vi "Drive Controller.vi"(8 "error in":errorcluster) -> ()   [LabVIEW 2018]
doc: "This VI executes continuously carrying out the current operation and responding to updates or new operation requests. It will often contain the timing or control code that is difficult to place directly in TeleOp. This VI generally opens all sensors and motors and isolates the rest of the robot code from knowing implementation details of how the operations are carried out."
uses:
  <vilib>/Rock Robotics/WPI/Framework/Completion Status.ctl
  Drive Setpoints.ctl
  Drive Operations.ctl
  <vilib>/Rock Robotics/SystemInterfaces/DIO/FPGA_DIOPWMChannel.ctl
  <vilib>/Rock Robotics/WPI/DriverStation/WPI_DriverStationRobotMode2.ctl
  <vilib>/Rock Robotics/WPI/RobotDrive/WPI_RobotDriveOpen4MotorWithJaguar.vi
  Framework/Robot Global Data.vi
  <vilib>/Rock Robotics/WPI/ThirdParty/Sensors/navX/_Processing Loop/FRIC_navX_Internal_SPI_ProcessingLoop.vi
panel:
  in  "Reset Gyro":bool
  in  "navX  start":dbl
  in  "Angle":dbl
  in  "Interactive Values":T1
  in  "Buttons":cluster{"Execute Cmd":bool, "Abort Cmd":bool}
  out "Command Timing":cluster{"Start Time (ms)":u32, "Iterations":i32}
  out "Status":T3
  out "Setpoints":T4(graph)
  out "Current\nCmd":string
  # "Tip: The graph shows the motor setpoints. It may also be helpful to observe inputs and sensor values.\nYou may also want to display tuning or debugging controls."
  # "Interactive Command: You may fill in the settings for a command\nand schedule it with the Execute button. You can observe and abort\nany command while fine tuning the code for the controller."
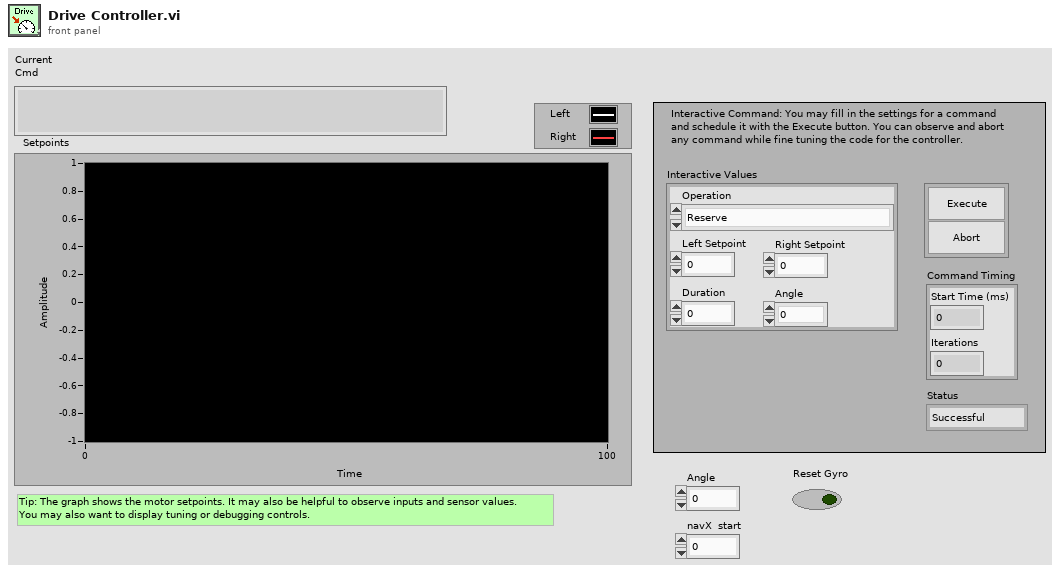
[diagram p1: front panel]
types:
  T1 = typedef "Drive Setpoints.ctl" = cluster{"Operation":T2, "Left Setpoint":dbl, "Right Setpoint":dbl, "Duration":dbl, "Angle":dbl}
  T2 = typedef "Drive Operations.ctl" = enum16{"Reserve", "Read Current", "Immediate", "Drive for Time", "Drive for Distance", "Turn to Angle"}
  T3 = typedef "Completion Status.ctl" = enum16{"Successful", "Aborted", "Incomplete"}
  T4 = cluster{"Left Setpoint":dbl, "Right Setpoint":dbl}
  T5 = typedef "FPGA_DIOPWMChannel.ctl" = enum8{"PWM 0", "PWM 1", "PWM 2", "PWM 3", "PWM 4", "PWM 5", "PWM 6", "PWM 7", "PWM 8", "PWM 9", "PWM MXP 0", "PWM MXP 1", "PWM MXP 2", "PWM MXP 3", "PWM MXP 4", "PWM MXP 5", "PWM MXP 6", "PWM MXP 7", "PWM MXP 8", "PWM MXP 9", "Invalid"}
  T6 = typedef "WPI_RobotDriveDevRef.ctl" = cluster{"DevStatus":errorcluster, "Motors[]":T7[], "Square Inputs":bool, "Max Output":dbl}
  T7 = typedef "WPI_MotorControlDeviceRef.ctl" = cluster{"DeviceStatus":errorcluster, "Type":T8, "PWM":cluster{"PWM Channel":T5, "DeadBand":T9}, "CAN":cluster{"Device Number":u8, "SetOutput VI Ref":variant, "GetOutput VI Ref":variant, "Enable VI Ref":variant, "Disable VI Ref":variant, "Data":variant}, "Invert":bool, "DIO PWM":cluster{"PWM \"Enable\" Channel":T5, "DIOChannel":T10, "PWM Rate":dbl}}
  T8 = typedef "WPI_MotorControlType.ctl" = enum16{"PWM", "CAN", "DIO PWM"}
  T9 = typedef "WPI_PWMDeadband.ctl" = cluster{"Name":string, "maxPositivePwm":i32, "minPositivePwm":i32, "centerPwm":i32, "maxNegativePwm":i32, "minNegativePwm":i32, "angularRange":u16}
  T10 = typedef "FPGA_DIOChannel.ctl" = enum8{"DIO 0", "DIO 1", "DIO 2", "DIO 3", "DIO 4", "DIO 5", "DIO 6", "DIO 7", "DIO 8", "DIO 9", "DIO MXP 0", "DIO MXP 1", "DIO MXP 2", "DIO MXP 3", "DIO MXP 4", "DIO MXP 5", "DIO MXP 6", "DIO MXP 7", "DIO MXP 8", "DIO MXP 9", "DIO MXP 10", "DIO MXP 11", "DIO MXP 12", "DIO MXP 13", "DIO MXP 14", "DIO MXP 15", "SPI Port CS1", "SPI Port CS2", "SPI Port CS3", "SPI Port MISO", "SPI Port MOSI", "Invalid"}
  T11 = typedef "Command Status Info.ctl" = cluster{"Name":string, "Status":T3, "notifier out":T12}
  T12 = typedef "Completion Notifier.ctl" = refnum<notifier>
  T13 = cluster{"SubSystem Data":T1, cluster{"Start Time (ms)":u32, "Iterations":i32}, cluster{"Command Info":T11, "Description":string, "Default Command":T1, "queue out":refnum<queue>, "Subsystem Name":string}}
  T14 = typedef "WPI_DriverStationRobotMode2.ctl" = enum16{"Autonomous Disabled", "Autonomous Enabled", "Teleop Disabled", "Teleop Enabled", "Disconnected", "Finish", "Test Disabled", "Test Enabled", "Emergency Stopped"}
  T15 = cluster{"Yaw":dbl, "Roll":dbl, "Pitch":dbl, "Heading":dbl, "Fused Heading":dbl}
  T16 = cluster{"SubSystem Data":T1, cluster{"Start Time (ms)":u32, "Iterations":i32}, "Default Command Arguments":cluster{"Command Info":T11, "Description":string, "Default Command":T1, "queue out":refnum<queue>, "Subsystem Name":string}}
  T17 = cluster{"Don't move motors while reserved":dbl, "Don't move motors while reserved":dbl}
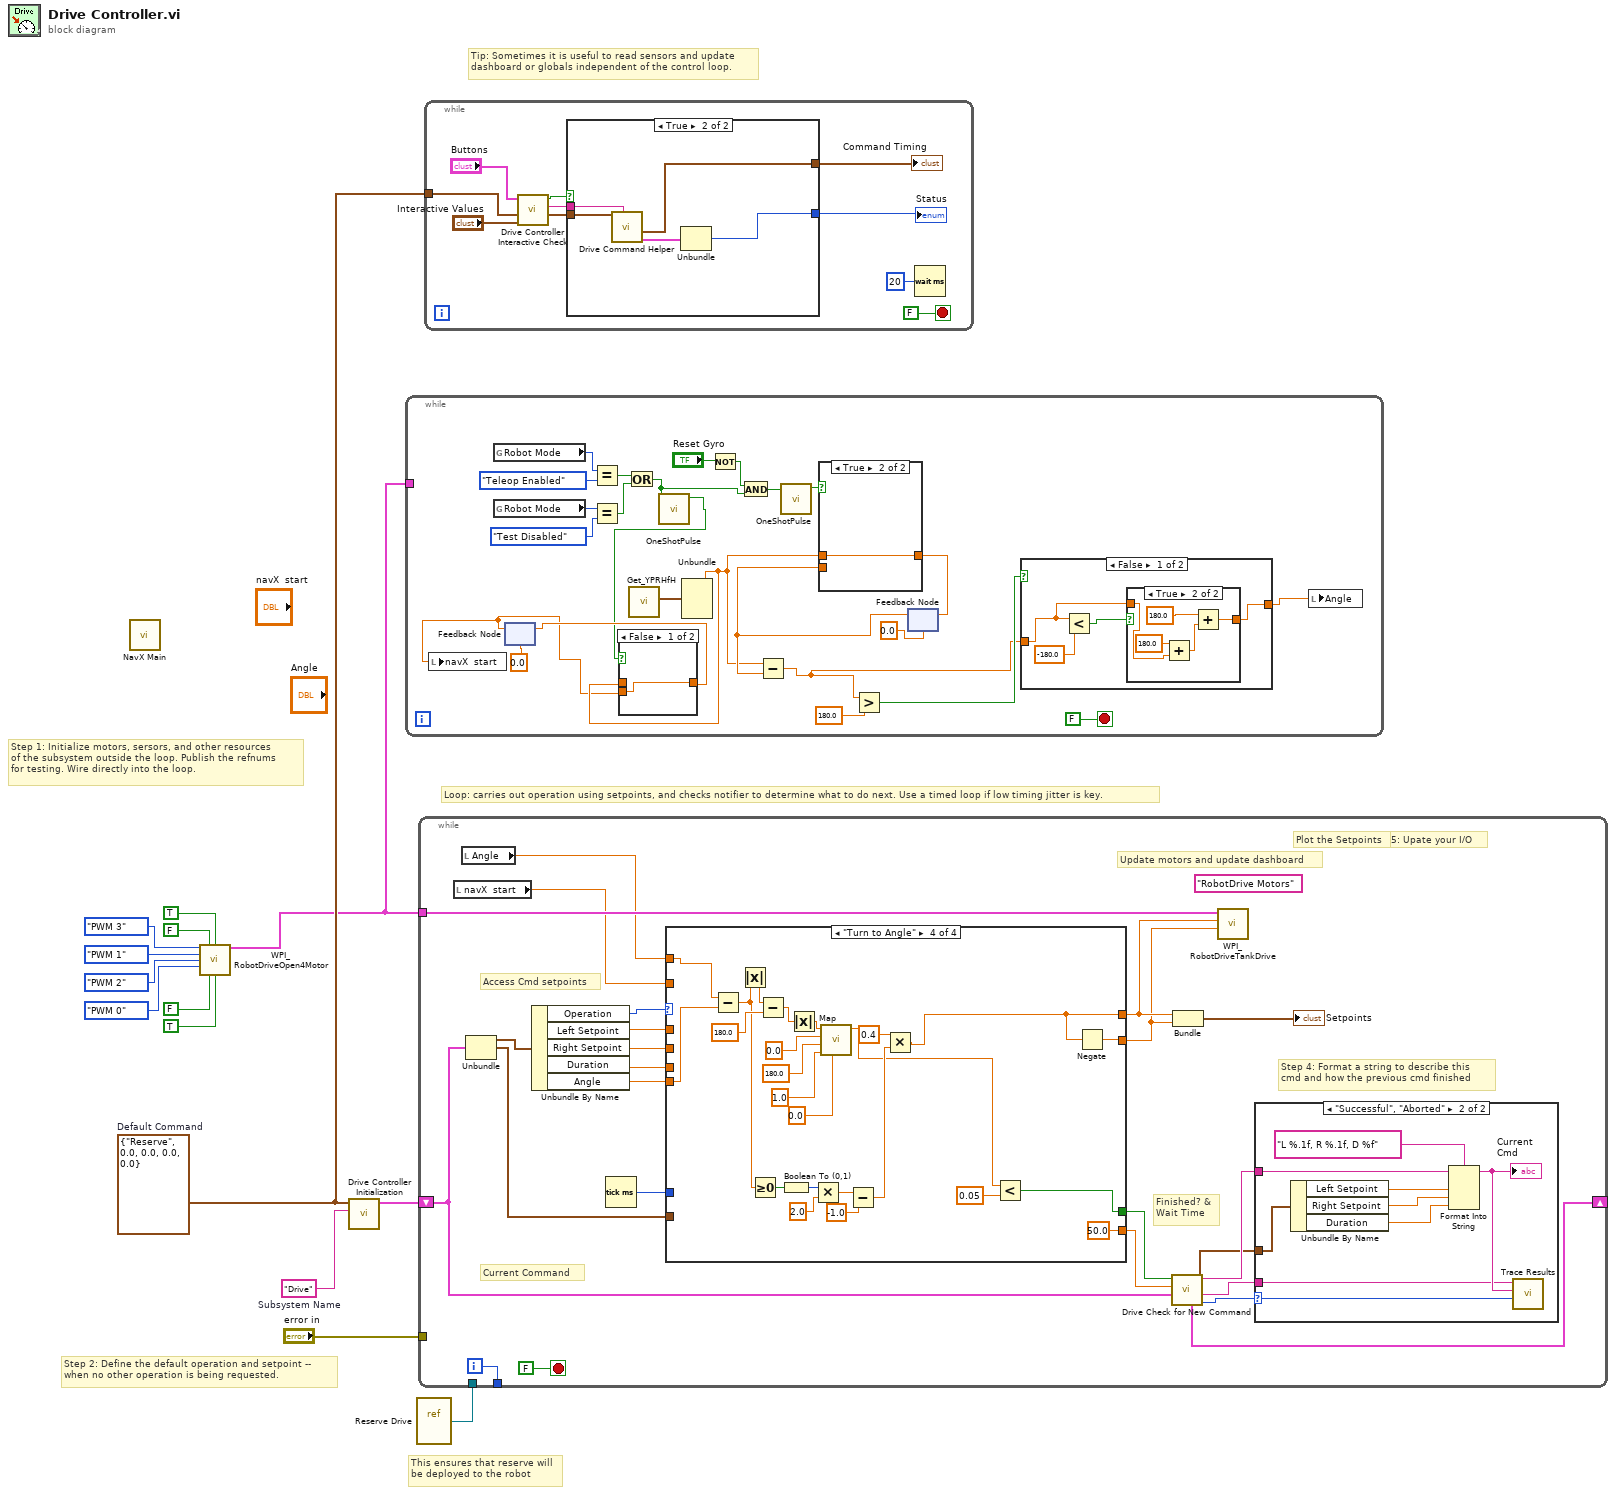
[diagram p0: block diagram]
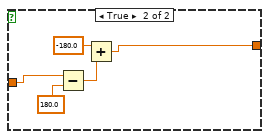
[diagram p3: hidden frame]
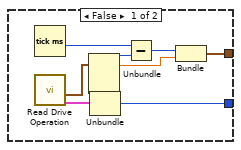
[diagram p6: hidden frame]
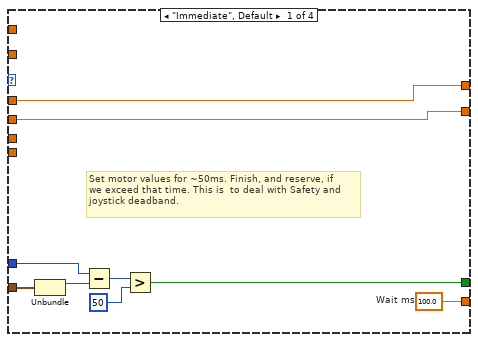
[diagram p8: hidden frame]
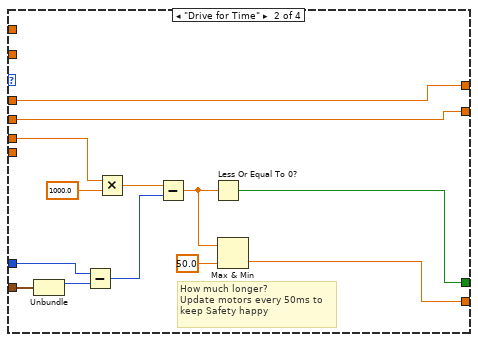
[diagram p9: hidden frame]
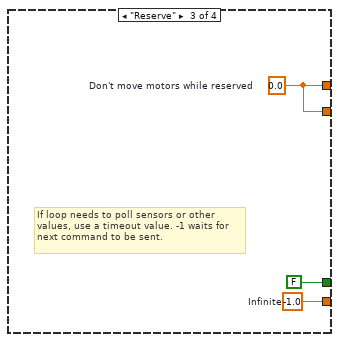
[diagram p10: hidden frame]
diagram:
  w10 = T1 {"Operation"=enum."Reserve", "Left Setpoint"=0.0, "Right Setpoint"=0.0, "Duration"=0.0, "Angle"=0.0}  # Default Command
  w14 = "Drive"  # Subsystem Name
  # "This ensures that reserve will\nbe deployed to the robot"
  # "Tip: Sometimes it is useful to read sensors and update\ndashboard or globals independent of the control loop."
  # "Step 2: Define the default operation and setpoint --\nwhen no other operation is being requested."
  # "Step 1: Initialize motors, sersors, and other resources\nof the subsystem outside the loop. Publish the refnums\nfor testing. Wire directly into the loop."
  # "Loop: carries out operation using setpoints, and checks notifier to determine what to do next. Use a timed loop if low timing jitter is key."
  n1 = call-poly <vilib>:"NavX Main.vi"() -> ()  [unwired: 12 in]
  n2 = call-poly <vilib>:"WPI_RobotDriveOpen4Motor.vi"("Rear Left Motor"=FPGA_DIOPWMChannel."PWM 3", "Rear Left Motor Inverted"=FALSE, "Rear Right Motor Inverted"=TRUE, "Rear Right Motor"=FPGA_DIOPWMChannel."PWM 1", "Front Left Motor"=FPGA_DIOPWMChannel."PWM 2", "Front Right Motor"=FPGA_DIOPWMChannel."PWM 0", "Front Left Motor Inverted"=FALSE, "Front Right Motor Inverted"=TRUE) -> ("RobotDriveDevRef"=w1:T6)  [unwired: 6 in, 1 out]
  n3 = call "Drive Controller Initialization.vi"("Subsystem Name"=w14, "Default Command"=w10) -> ("Current Command"=w12:T13)  [unwired: 9 in]
  n4 = while {
    tunnel: w1 -> [_]
    stop <- FALSE stop-if-true
    n5 = global read "Robot Global Data.vi" "Robot Mode"() -> (w35:T14)
    n6 = global read "Robot Global Data.vi" "Robot Mode"() -> (w37:T14)
    n7 = feedback #1(0.0) -> (w25:dbl)
    n8 = local write "navX  start"(w25) -> ()
    n9 = Equal?(x=w35, y=WPI_DriverStationRobotMode2."Teleop Enabled") -> (x = y?=w33:bool)
    n10 = Equal?(x=w37, y=WPI_DriverStationRobotMode2."Test Disabled") -> (x = y?=w32:bool)
    n11 = Or(x=w33, y=w32) -> (x .or. y?=w19:bool)
    n12 = call <vilib>:"Get_YPRHfH.vi"() -> ("YRPHfH"=w38:T15)  [unwired: 11 in]
    n13 = call "OneShotPulse.vi"("Input"=w19) -> ("Output"=w24:bool)  [unwired: 10 in]
    n14 = Unbundle(w38) -> ("Yaw"=w27:dbl)  [unwired: 4 out]
    n15 = case shown="False" w24 {
      tunnel: w27 -> [_ w56]
      tunnel: [w55 w56] -> w26
      tunnel: w25 -> [w55 _]
      frame False {
      }
      frame True {
      }
    }
    n16 = feedback-in #1(w26) -> ()
    n17 = Not(x="Reset Gyro") -> (.not. x?=w20:bool)
    n18 = And(x=w20, y=w19) -> (x .and. y?=w22:bool)
    n19 = call "OneShotPulse.vi"("Input"=w22) -> ("Output"=w23:bool)  [unwired: 10 in]
    n20 = feedback #2(0.0 ("Yaw")) -> (w29:dbl)
    n21 = Subtract(x=w27, y=w29) -> (x-y=w15:dbl)
    n22 = case shown="True" w23 {
      tunnel: w27 -> [_ w58]
      tunnel: [w57 w58] -> w31
      tunnel: w29 -> [w57 _]
      frame False {
      }
      frame True {
      }
    }
    n23 = Greater?(x=w15, y=180.0) -> (0:w17:bool)
    n24 = feedback-in #2(w31) -> ()
    n25 = case shown="False" w17 {
      tunnel: [w40 w52] -> w16
      tunnel: w15 -> [w41 w50]
      frame False {
        n26 = Less?(x=w41, y=-180.0) -> (x < y?=w42:bool)
        n27 = case shown="True" w42 {
          tunnel: w41 -> [w44 w47]
          tunnel: [w44 w45] -> w40
          frame False {
          }
          frame True {
            n28 = Add(x=180.0, y=w47) -> (x+y=w46:dbl)
            n29 = Add(x=180.0, y=w46) -> (x+y=w45:dbl)
          }
        }
      }
      frame True {
        n30 = Subtract(x=w50, y=180.0) -> (x-y=w53:dbl)
        n31 = Add(x=-180.0, y=w53) -> (x+y=w52:dbl)
      }
    }
    n32 = local write "Angle"(w16) -> ()
  }
  n33 = vi-ref "Reserve Drive.vi"() -> (w11:refnum<vi>)
  n34 = while {
    shift-right: [w69] -> _
    shift-left: w12 -> [w62]
    tunnel: [w81] -> _
    tunnel: w1 -> [w77]
    tunnel: "error in" -> [_]
    tunnel: w11 -> [_]
    i -> [w81]
    stop <- FALSE stop-if-true
    (unwired) "RobotDrive Motors" ("Name")
    # "Step 5: Upate your I/O"
    # "Step 4: Format a string to describe this\ncmd and how the previous cmd finished"
    # "Current Command"
    # "Update motors and update dashboard"
    # "Plot the Setpoints"
    # "Access Cmd setpoints"
    # "Finished? &\nWait Time"
    n35 = local read "navX  start"() -> (w59:dbl)
    n36 = local read "Angle"() -> (w60:dbl)
    n37 = Unbundle(w62) -> ("SubSystem Data"=w76:T1, w63:cluster{"Start Time (ms)":u32, "Iterations":i32})  [unwired: 1 out]
    n38 = Unbundle By Name(w76) -> ("Operation"=w75:T2, "Left Setpoint"=w74:dbl, "Right Setpoint"=w73:dbl, "Duration"=w72:dbl, "Angle"=w61:dbl)
    n39 = Tick Count (ms)() -> (millisecond timer value=w71:u32)
    n40 = case shown="\"Turn to Angle\"" w75 {
      tunnel: [w100 w101 w116 50.0 ("Infinite")] -> w68
      tunnel: [w93 w108 FALSE ("ignore previous (F)") w138] -> w67
      tunnel: w63 -> [w92 w110 _ _]
      tunnel: [w99 w107 w114 w136] -> w79
      tunnel: [w98 w106 w114 w137] -> w78
      tunnel: w74 -> [w99 w107 _ _]
      tunnel: w73 -> [w98 w106 _ _]
      tunnel: w72 -> [_ w105 _ _]
      tunnel: w71 -> [w94 w104 _ _]
      tunnel: w60 -> [_ _ _ w118]
      tunnel: w61 -> [_ _ _ w135]
      tunnel: w59 -> [_ _ _ _]
      frame "Immediate", Default {
        w100 = 100.0  # Wait ms
        # "Set motor values for ~50ms. Finish, and reserve, if\nwe exceed that time. This is  to deal with Safety and\njoystick deadband."
        n41 = Unbundle(w92) -> ("Start Time (ms)"=w95:u32)  [unwired: 1 out]
        n42 = Subtract(x=w94, y=w95) -> (x-y=w96:u32)
        n43 = Greater?(x=w96, y=u8 50 ("Left Motor")) -> (0:w93:bool)
      }
      frame "Drive for Time" {
        # "How much longer?\nUpdate motors every 50ms to\nkeep Safety happy"
        n44 = Unbundle(w110) -> ("Start Time (ms)"=w109:u32)  [unwired: 1 out]
        n45 = Subtract(x=w104, y=w109) -> (x-y=w113:u32)
        n46 = Multiply(x=w105, y=1000.0) -> (x*y=w112:dbl)
        n47 = Subtract(x=w112, y=w113) -> (x-y=w103:dbl)
        n48 = Less Or Equal To 0?(x=w103) -> (x <= 0?=w108:bool)
        n49 = Max & Min(x=w103, y=50.0) -> (min(x,y)=w101:dbl)  [unwired: 1 out]
      }
      frame "Reserve" {
        w114 = 0.0  # Don't move motors while reserved
        w116 = -1.0  # Infinite
        # "If loop needs to poll sensors or other\nvalues, use a timeout value. -1 waits for\nnext command to be sent."
      }
      frame "Turn to Angle" {
        n50 = Subtract(x=w118, y=w135) -> (x-y=w126:dbl)
        n51 = Absolute Value(x=w126) -> (abs(x)=w127:dbl)
        n52 = Greater Or Equal To 0?(x=w126) -> (x >= 0?=w125:bool)
        n53 = Subtract(x=w127, y=180.0) -> (x-y=w128:dbl)
        n54 = Boolean To (0,1)(Boolean=w125) -> (0, 1=w124:i16)
        n55 = Absolute Value(x=w128) -> (abs(x)=w134:dbl)
        n56 = Multiply(x=w124, y=2.0) -> (x*y=w122:dbl)
        n57 = call "Map.vi"("B max"=0.0, "B min"=1.0, "A max"=180.0, "A min"=0.0, "A"=w134) -> ("B"=w117:dbl)  [unwired: 6 in]
        n58 = Subtract(x=w122, y=-1.0) -> (x-y=w120:dbl)
        n59 = Multiply(x=0.4, y=w120) -> (x*y=w136:dbl)
        n60 = Less?(x=w117, y=0.05) -> (x < y?=w138:bool)
        n61 = Negate(x=w136) -> (-x=w137:dbl)
      }
    }
    n62 = call "Drive Check for New Command.vi"("input cluster"=w62, "Wait time (ms)"=w68, "Finished?"=w67) -> ("Completion"=w70:T3, "Subsystem Name"=w64:string, "Current Command"=w65:T1, "Initial Trace String"=w66:string, "Next Command"=w69:T16)  [unwired: 4 in]
    n63 = Bundle("Don't move motors while reserved"=w79, "Don't move motors while reserved"=w78) -> (→"Setpoints":T17)  [unwired: 1 in]
    n64 = call <vilib>:"WPI_RobotDriveTankDrive.vi"("Right axis value"=w78, "Left axis value"=w79, "RobotDriveDevRef"=w77) -> ()  [unwired: 6 in, 3 out]
    n65 = case shown="\"Successful\", \"Aborted\"" w70 {
      selector: w70 -> [_ w91]
      tunnel: w66 -> [_ w86]
      tunnel: w65 -> [_ w87]
      tunnel: w64 -> [_ w83]
      frame "Incomplete", Default {
        # "Continuing current command"
      }
      frame "Successful", "Aborted" {
        # "Report and setup for next command"
        n66 = Unbundle By Name(w87) -> ("Left Setpoint"=w89:dbl, "Right Setpoint"=w90:dbl, "Duration"=w84:dbl)
        n67 = Format Into String(format string="L %.1f, R %.1f, D %f", initial string=w86, w89, w90, w84) -> (resulting string=w85:string)  [unwired: 1 in, 1 out]
        "Current\nCmd" <- w85
        n68 = call <vilib>:"Trace Results.vi"("Status of previous command"=w91, "Description"=w85, "Subsystem"=w83) -> ()  [unwired: 9 in]
      }
    }
  }
  n69 = while {
    tunnel: w10 -> [w142]
    stop <- FALSE stop-if-true
    n70 = call "Drive Controller Interactive Check.vi"("Interactive Command In"="Interactive Values", "Default Command"=w142, "Buttons"="Buttons") -> ("Interactive Command Out"=w144:T1, "Trace String"=w145:string, "Schedule"=w146:bool)  [unwired: 6 in]
    n71 = case shown="True" w146 {
      tunnel: [w155 w163] -> w147
      tunnel: [w154 w159] -> w148
      tunnel: w145 -> [_ w161]
      tunnel: w144 -> [_ w160]
      frame False {
        n72 = Tick Count (ms)() -> (millisecond timer value=w158:u32)
        n73 = call "Read Drive Operation.vi"() -> ("Command Info"=w152:T11, "SubSystem Data"=w151:T1)  [unwired: 9 in, 1 out]
        n74 = Unbundle(w151) -> ("Operation"=w156:T2, "Left Setpoint"=w153:dbl)  [unwired: 3 out]
        n75 = Unbundle(w152) -> ("Status"=w155:T3)  [unwired: 2 out]
        n76 = Subtract(x=w158, y=w156) -> (x-y=w157:u32)
        n77 = Bundle(w157, "Left Setpoint"=w153) -> (w154:cluster{u32, "Left Setpoint":dbl})  [unwired: 1 in]
      }
      frame True {
        n78 = call "Drive Command Helper.vi"("Description"=w161, "SubSystem Data"=w160) -> ("Command Info Out"=w162:T11, "Command Timing"=w159:cluster{"Start Time (ms)":u32, "Iterations":i32})  [unwired: 7 in, 1 out]
        n79 = Unbundle(w162) -> ("Status"=w163:T3)  [unwired: 2 out]
      }
    }
    "Status" <- w147
    "Command Timing" <- w148
    n80 = Wait (ms)(milliseconds to wait=u32 20) -> ()  [unwired: 1 out]
  }
